vi "setIDs.vi"(8 "error in (no error)":errorcluster, 9 "Nodes in":refnum<data-value>[](array[refnum]), 10 "IDs in":u32[](array[numeric]), 11 "GraphNode in":refnum<class "GraphNode.lvclass">) -> (0 "error out":errorcluster, 1 "Nodes out":refnum<data-value>[](array[refnum]), 2 "IDs out":u32[](array[numeric]), 3 "GraphNode out":refnum<class "GraphNode.lvclass">)   [LabVIEW 2009, in "GraphNode.lvclass"]
uses:
  GraphNode.lvclass
  DataObj/DataObj.lvclass
  Node/Node.lvclass
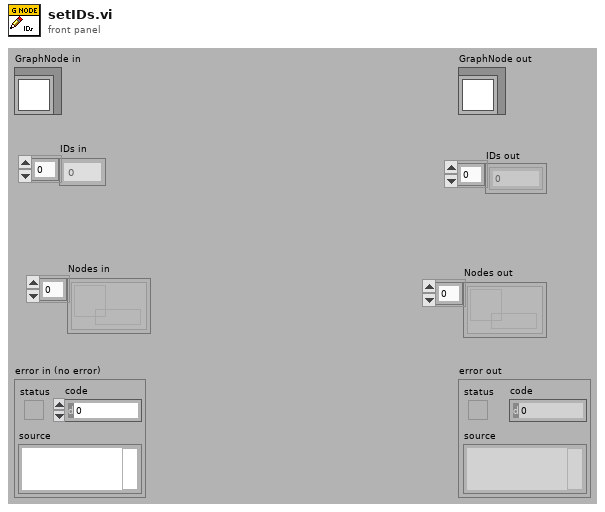
[diagram p1: front panel]
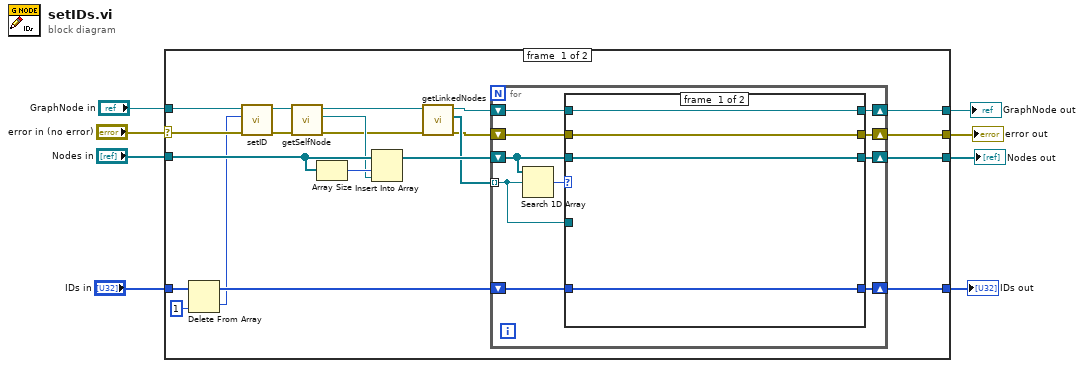
[diagram p0: block diagram]
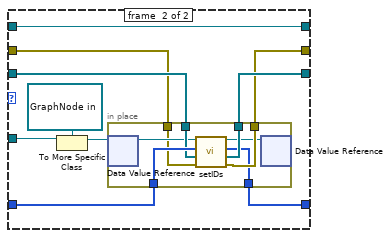
[diagram p2: hidden frame]
diagram:
  n1 = case shown="No Error" "error in (no error)" {
    selector: "error in (no error)" -> [w14 w65]
    tunnel: [w18 w65] -> w7
    tunnel: [w19 w64] -> w6
    tunnel: "GraphNode in" -> [w15 w64]
    tunnel: "Nodes in" -> [w28 w63]
    tunnel: [w20 w63] -> w3
    tunnel: "IDs in" -> [w13 w62]
    tunnel: [w9 w62] -> w1
    frame #0 {
      n2 = Delete From Array(array=w13, index=1) -> (deleted portion=w10:u32, array with subset deleted=w11:u32[])  [unwired: 1 in]
      n3 = call "setID.vi"("error in (no error)"=w14, "ID"=w10, "Node in"=w15) -> ("error out"=w16:errorcluster, "Node out"=w17:refnum<class "GraphNode.lvclass">)  [unwired: 7 in]
      n4 = call "getSelfNode.vi"("error in (no error)"=w16, "Node in"=w17) -> ("error out"=w25:errorcluster, "selfNode"=w27:refnum<data-value>, "Node out"=w26:refnum<class "GraphNode.lvclass">)  [unwired: 7 in]
      n5 = Array Size(array=w28) -> (size(s)=w29:i32)
      n6 = Insert Into Array(array=w28, index=w29, new element=w27) -> (w24:refnum<data-value>[])
      n7 = call "getLinkedNodes.vi"("error in (no error)"=w25, "GraphNode in"=w26) -> ("error out"=w22:errorcluster, "LinkedNodes"=w23:refnum<data-value>[], "GraphNode out"=w21:refnum<class "GraphNode.lvclass">)  [unwired: 7 in]
      n8 = for {
        tunnel: w23 -> [w38] mode=indexing
        shift-right: [w32] -> w18
        shift-left: w22 -> [w33]
        shift-right: [w36] -> w19
        shift-left: w21 -> [w37]
        shift-right: [w34] -> w20
        shift-left: w24 -> [w35]
        shift-right: [w30] -> w9
        shift-left: w11 -> [w31]
        n9 = Search 1D Array(1D array=w35, element=w38) -> (index of element=w39:i32)  [unwired: 1 in]
        n10 = case shown="-1" w39 {
          tunnel: w38 -> [_ w53]
          tunnel: w37 -> [w43 w50]
          tunnel: [w43 w50] -> w36
          tunnel: w35 -> [w42 w49]
          tunnel: [w42 w48] -> w34
          tunnel: w33 -> [w41 w47]
          tunnel: [w41 w46] -> w32
          tunnel: w31 -> [w40 w45]
          tunnel: [w40 w44] -> w30
          frame #0 {
          }
          frame #1 {
            n11 = To More Specific Class(target class=refnum<data-value> refnum ("data value reference"), reference=w53) -> (specific class reference=w51:refnum<data-value>)  [unwired: 1 in, 1 out]
            n12 = in-place {
              in-place-border: w49 -> [w60]
              in-place-border: [w59] -> w48
              in-place-border: w47 -> [w55]
              in-place-border: [w58] -> w46
              in-place-border: w45 -> [w61]
              in-place-border: [w54] -> w44
              n13 = in-place-dvr #1(w51) -> (w57:refnum<class "GraphNode.lvclass">)  [unwired: 1 out]
              n14 = call "setIDs.vi"("error in (no error)"=w55, "Nodes in"=w60, "IDs in"=w61, "GraphNode in"=w57) -> ("error out"=w58:errorcluster, "Nodes out"=w59:refnum<data-value>[], "IDs out"=w54:u32[], "GraphNode out"=w56:refnum<class "GraphNode.lvclass">)  [unwired: 4 in]
              n15 = in-place-dvr #1(w56) -> ()  [unwired: 2 out]
            }
          }
        }
      }
    }
    frame #1 {
    }
  }
  "error out" <- w7
  "GraphNode out" <- w6
  "Nodes out" <- w3
  "IDs out" <- w1
